vi "Configure Test CRDS.vi"(8 "error in (no error)":errorcluster, 11 "CRDS in":refnum<class "CRDS.lvclass">) -> (0 "error out":errorcluster, 3 "CRDS out":refnum<class "CRDS.lvclass">)   [LabVIEW 2015, in "CRDS.lvclass"]
uses:
  Main/CRDS.lvclass
  Cell/CRDS Cell.lvclass
  Data/Cell/CRDS Cell Data.lvclass
  Cell/Get Tau Method.ctl
  General/Math/Fit Exponential Class/Children/LRS/LRS.lvclass
  Data/Main/CRDS Data.lvclass
  Cell/CRDS Cell.lvclass/CRDS Cell.ctl
  Main/CRDS.lvclass/CRDS.ctl
  Cell/Write Data.vi
  Cell/Write ExpFit.vi
  Cell/Write Nremove.vi
  Main/Write NumCoadd.vi
  General/Atmospheric/Atmospheric Constants.vi
  Cell/Write CalType.vi
  Cell/Write dt.vi
  Cell/Write errorCalOn.vi
  Cell/Write optTimeConst.vi
  Cell/Write lambda.vi
  Data/Main/Write CellData.vi
  Main/Write Cells.vi
  Main/Write Data.vi
  Main/Write goodData.vi
  General/Atmospheric/Atmospheric Library.lvlib
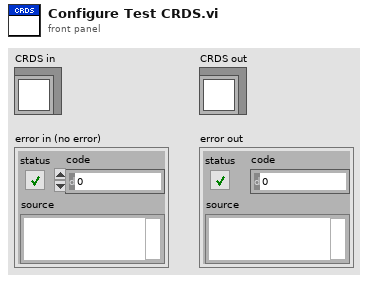
[diagram p1: front panel]
types:
  T1 = typedef "Get Tau Method.ctl" = enum8{"DFT-1", "DFT-5", "LRS"}
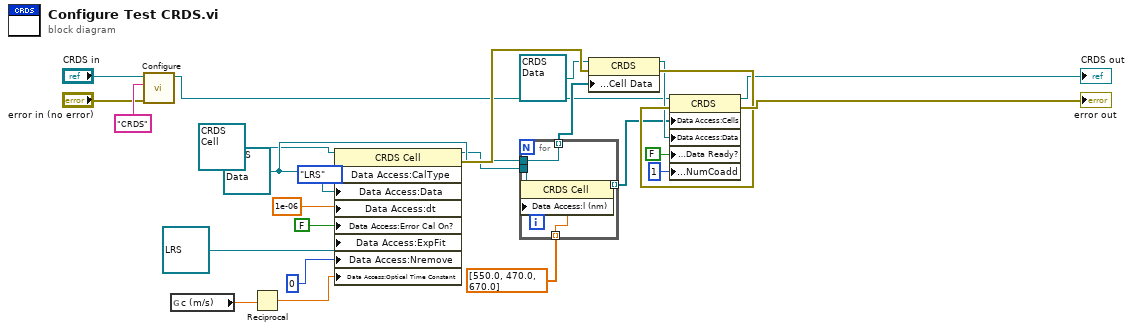
[diagram p0: block diagram]
diagram:
  w18 = refnum<class "CRDS Cell Data.lvclass"> refnum ("Data")
  n1 = call-dynamic "Configure.vi"("error in"="error in (no error)", "name"="CRDS", "CRDS in"="CRDS in") -> ("CRDS out"=w14:refnum<class "CRDS.lvclass">)  [unwired: 7 in, 1 out]
  n2 = global read "Atmospheric Constants.vi" "c (m/s)"() -> (w10:dbl)
  n3 = Reciprocal(x=w10) -> (1/x=w11:dbl)
  n4 = property class="CRDS Cell"(reference=refnum<class "CRDS Cell.lvclass"> refnum ("CRDS Cell"), "Data Access:CalType"=Get_Tau_Method."LRS" ("CalType"), "Data Access:Data"=w18, "Data Access:dt"=1e-06 ("dt"), "Data Access:Error Cal On?"=FALSE ("Error Cal On?"), "Data Access:ExpFit"=refnum<class "LRS.lvclass"> refnum ("Exponential Fit Lib:LRS"), "Data Access:Nremove"=0 ("Nremove"), "Data Access:Optical Time Constant"=w11) -> (reference out=w12:refnum<class "CRDS Cell.lvclass">, error out=w23:errorcluster)  [unwired: 1 in]
  n5 = for {
    tunnel: w12 -> [w29]
    tunnel: dbl[] [550.0, 470.0, 670.0] -> [w28] mode=indexing
    tunnel: [w27] -> w15 mode=indexing
    tunnel: w18 -> [w26]
    tunnel: [w26] -> w20 mode=indexing
    n6 = property class="CRDS Cell"(reference=w29, "Data Access:l (nm)"=w28) -> (reference out=w27:refnum<class "CRDS Cell.lvclass">)  [unwired: 1 in, 1 out]
  }
  n7 = property class="CRDS"(reference=refnum<class "CRDS Data.lvclass"> refnum ("CRDS"), error in=w23, "Data Access:Cell Data"=w20) -> (reference out=w21:refnum<class "CRDS Data.lvclass">, error out=w24:errorcluster)
  n8 = property class="CRDS"(reference=w14, error in=w24, "Data Access:Cells"=w15, "Data Access:Data"=w21, "Data Access:Data Ready?"=FALSE ("Data Ready?"), "Accessors:NumCoadd"=1 ("NumCoadd")) -> (reference out=→"CRDS out":refnum<class "CRDS.lvclass">, error out=→"error out":errorcluster)
